vi "Second Graph Handler.vi"(0 "WF Ref Array":refnum<vi>[](array[refnum]), 2 "State":string, 7 "Data":dbl[](array[numeric]), 11 "CommandCluster":T1) -> ()   [LabVIEW 2019]
uses:
  TypeDef/Command Cluster.ctl
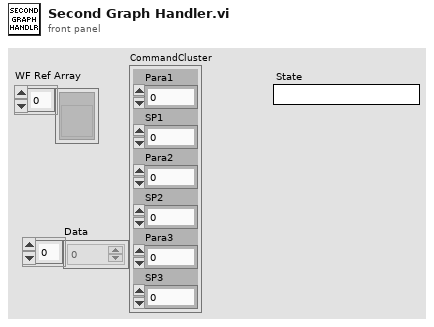
[diagram p1: front panel]
types:
  T1 = typedef "Command Cluster.ctl" = cluster{"Para1":i32, "SP1":dbl, "Para2":i32, "SP2":dbl, "Para3":i32, "SP3":dbl}
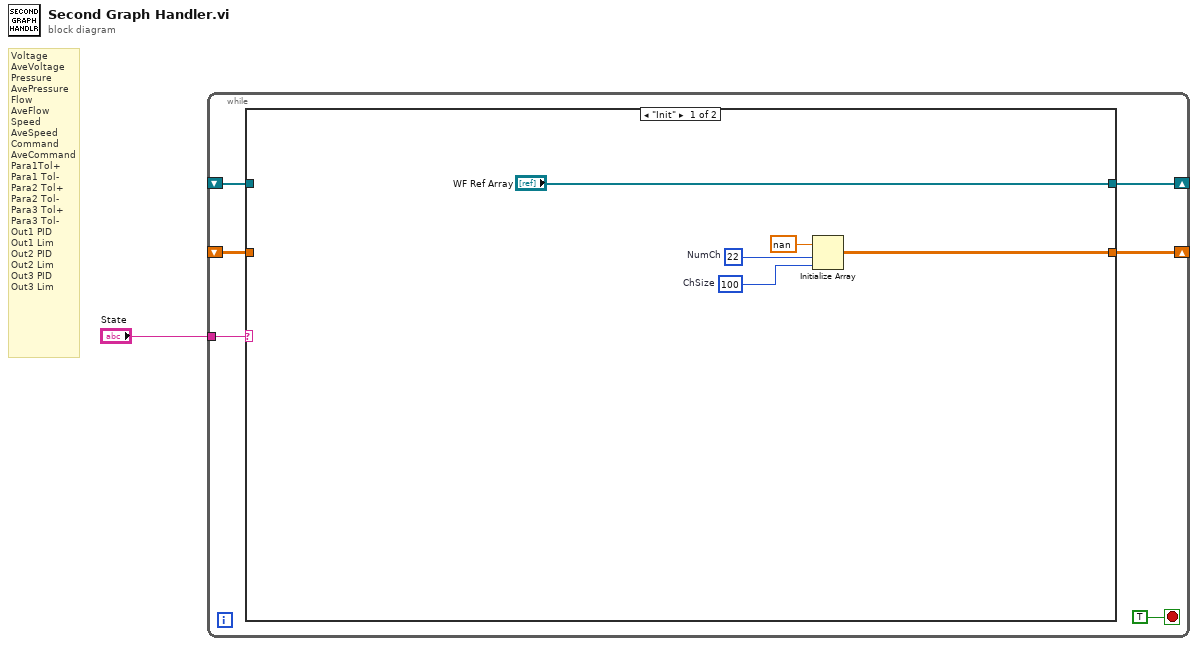
[diagram p0: block diagram]
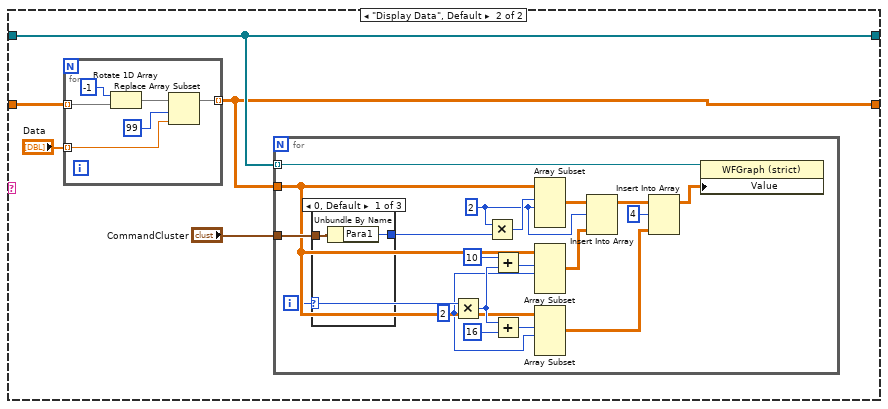
[diagram p2: hidden frame]
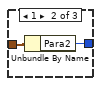
[diagram p3: hidden frame]
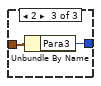
[diagram p4: hidden frame]
diagram:
  # "Voltage\nAveVoltage\nPressure\nAvePressure\nFlow\nAveFlow\nSpeed\nAveSpeed\nCommand\nAveCommand\nPara1Tol+\nPara1 Tol-\nPara2 Tol+\nPara2 Tol-\nPara3 Tol+\nPara3 Tol-\nOut1 PID\nOut1 Lim\nOut2 PID\nOut2 Lim\nOut3 PID\nOut3 Lim"
  n1 = while {
    tunnel: "State" -> [w6]
    shift-right: [w4] -> _
    shift-left: _ -> [w3]
    shift-right: [w5] -> _
    shift-left: _ -> [w2]
    stop <- TRUE stop-if-true
    n2 = case shown="\"Init\"" w6 {
      tunnel: [w12 w14] -> w5
      tunnel: ["WF Ref Array" w15] -> w4
      tunnel: w3 -> [_ w15]
      tunnel: w2 -> [_ w17]
      frame "Init" {
        w9 = 22  # NumCh
        w11 = 100  # ChSize
        n3 = Initialize Array(nan, w9, w11) -> (w12:dbl[][])
      }
      frame "Display Data", Default {
        n4 = for {
          tunnel: w17 -> [w47] mode=indexing
          tunnel: [w44] -> w14 mode=indexing
          tunnel: "Data" -> [w45] mode=indexing
          n5 = Rotate 1D Array(1:w47, 2:-1 ("n")) -> (0:w46:dbl[])
          n6 = Replace Array Subset(array=w46, new element=w45, index=99) -> (w44:dbl[])
        }
        n7 = for {
          tunnel: w15 -> [w22] mode=indexing
          tunnel: w14 -> [w21]
          tunnel: "CommandCluster" -> [w36]
          i -> [w20]
          w19 = 2 ("y")
          w24 = 2 ("length")
          n8 = case shown="0, Default" w20 {
            tunnel: w36 -> [w38 w40 w42]
            tunnel: [w37 w39 w41] -> w18
            frame 0, Default {
              n9 = Unbundle By Name(w38) -> ("Para1"=w37:i32)
            }
            frame 1 {
              n10 = Unbundle By Name(w40) -> ("Para2"=w39:i32)
            }
            frame 2 {
              n11 = Unbundle By Name(w42) -> ("Para3"=w41:i32)
            }
          }
          n12 = Multiply(x=w20, y=w19) -> (x*y=w30:i32)
          n13 = Multiply(x=w24, y=w18) -> (x*y=w25:i32)
          n14 = Add(x=10, y=w30) -> (x+y=w27:i32)
          n15 = Add(x=w30, y=16) -> (x+y=w26:i32)
          n16 = Array Subset(array=w21, index (row)=w25, length (row)=w24) -> (w35:dbl[][])  [unwired: 2 in]
          n17 = Array Subset(array=w21, index (row)=w27, length (row)=w19) -> (w31:dbl[][])  [unwired: 2 in]
          n18 = Array Subset(array=w21, index (row)=w26, length (row)=w19) -> (w32:dbl[][])  [unwired: 2 in]
          n19 = Insert Into Array(array=w35, index (row)=w24, new element=w31) -> (w34:dbl[][])  [unwired: 1 in]
          n20 = Insert Into Array(array=w34, index (row)=4, new element=w32) -> (w33:dbl[][])  [unwired: 1 in]
          n21 = property class="WFGraph (strict)"(reference=w22, "Value"=w33) -> ()  [unwired: 1 in, 2 out]
        }
      }
    }
  }
